vi "Read Escape URLs.vi"(8 "error in (no error)":errorcluster, 11 "REST Client in":refnum<class "REST Client.lvclass">) -> (0 "error out":errorcluster, 2 "Escape URLs":bool, 3 "REST Client out":refnum<class "REST Client.lvclass">)   [LabVIEW 2013, in "REST Client.lvlib" / "REST Client.lvclass"]
doc: "Read Escape URLs"
uses:
  REST Client.lvclass
  REST Client.lvclass/REST Client.ctl
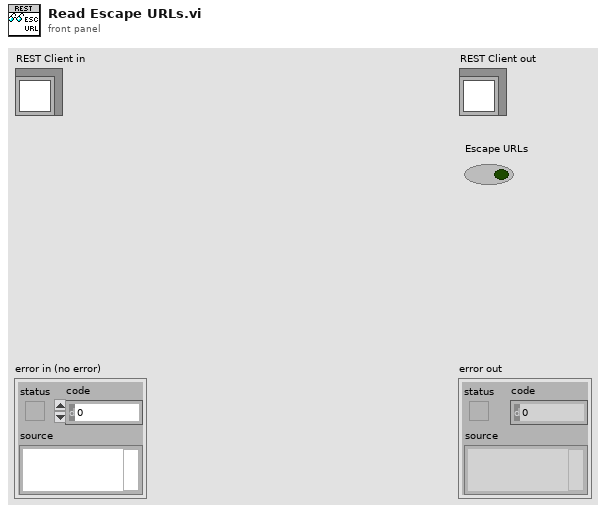
[diagram p1: front panel]
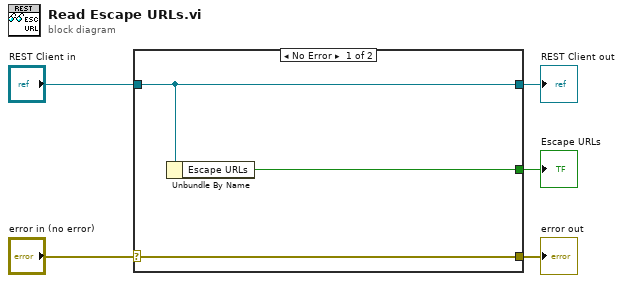
[diagram p0: block diagram]
diagram:
  n1 = case shown="No Error" "error in (no error)" {
    selector: "error in (no error)" -> [w8 w9]
    tunnel: [w8 w9] -> w4
    tunnel: [w7 w10] -> w2
    tunnel: "REST Client in" -> [w7 w10]
    tunnel: [w6 _] -> w1
    frame No Error {
      n2 = Unbundle By Name(w7) -> ("Escape URLs"=w6:bool)
    }
    frame Error {
    }
  }
  "error out" <- w4
  "REST Client out" <- w2
  "Escape URLs" <- w1
